vi "Updated Set Pointcycles.vi"(6 "Time2":T3, 8 "Time1":T2, 9 "rate":dbl, 10 "Amp":T1, 11 "i":i32) -> (12 "Gain times":cluster{dbl, dbl, dbl, dbl, dbl, dbl}, 13 "y":dbl)   [LabVIEW 2011]
panel:
  out "I tot":dbl
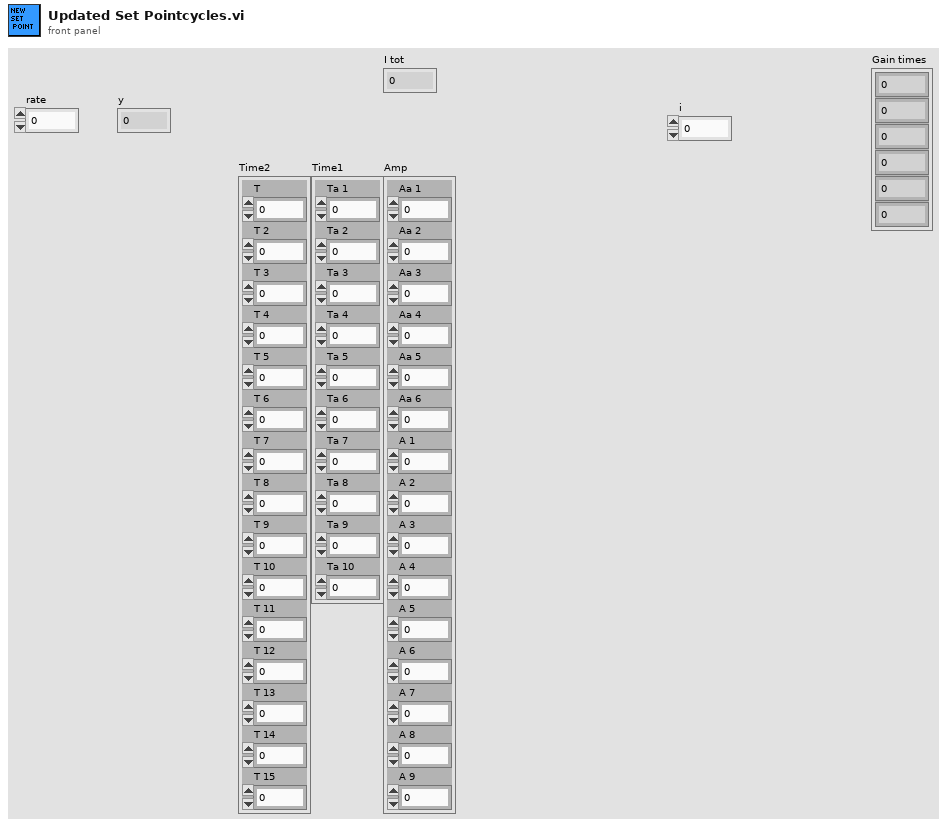
[diagram p1: front panel]
types:
  T1 = cluster{"Aa 1":dbl, "Aa 2":dbl, "Aa 3":dbl, "Aa 4":dbl, "Aa 5":dbl, "Aa 6":dbl, "A 1":dbl, "A 2":dbl, "A 3":dbl, "A 4":dbl, "A 5":dbl, "A 6":dbl, "A 7":dbl, "A 8":dbl, "A 9":dbl}
  T2 = cluster{"Ta 1":dbl, "Ta 2":dbl, "Ta 3":dbl, "Ta 4":dbl, "Ta 5":dbl, "Ta 6":dbl, "Ta 7":dbl, "Ta 8":dbl, "Ta 9":dbl, "Ta 10":dbl}
  T3 = cluster{"T":dbl, "T 2":dbl, "T 3":dbl, "T 4":dbl, "T 5":dbl, "T 6":dbl, "T 7":dbl, "T 8":dbl, "T 9":dbl, "T 10":dbl, "T 11":dbl, "T 12":dbl, "T 13":dbl, "T 14":dbl, "T 15":dbl}
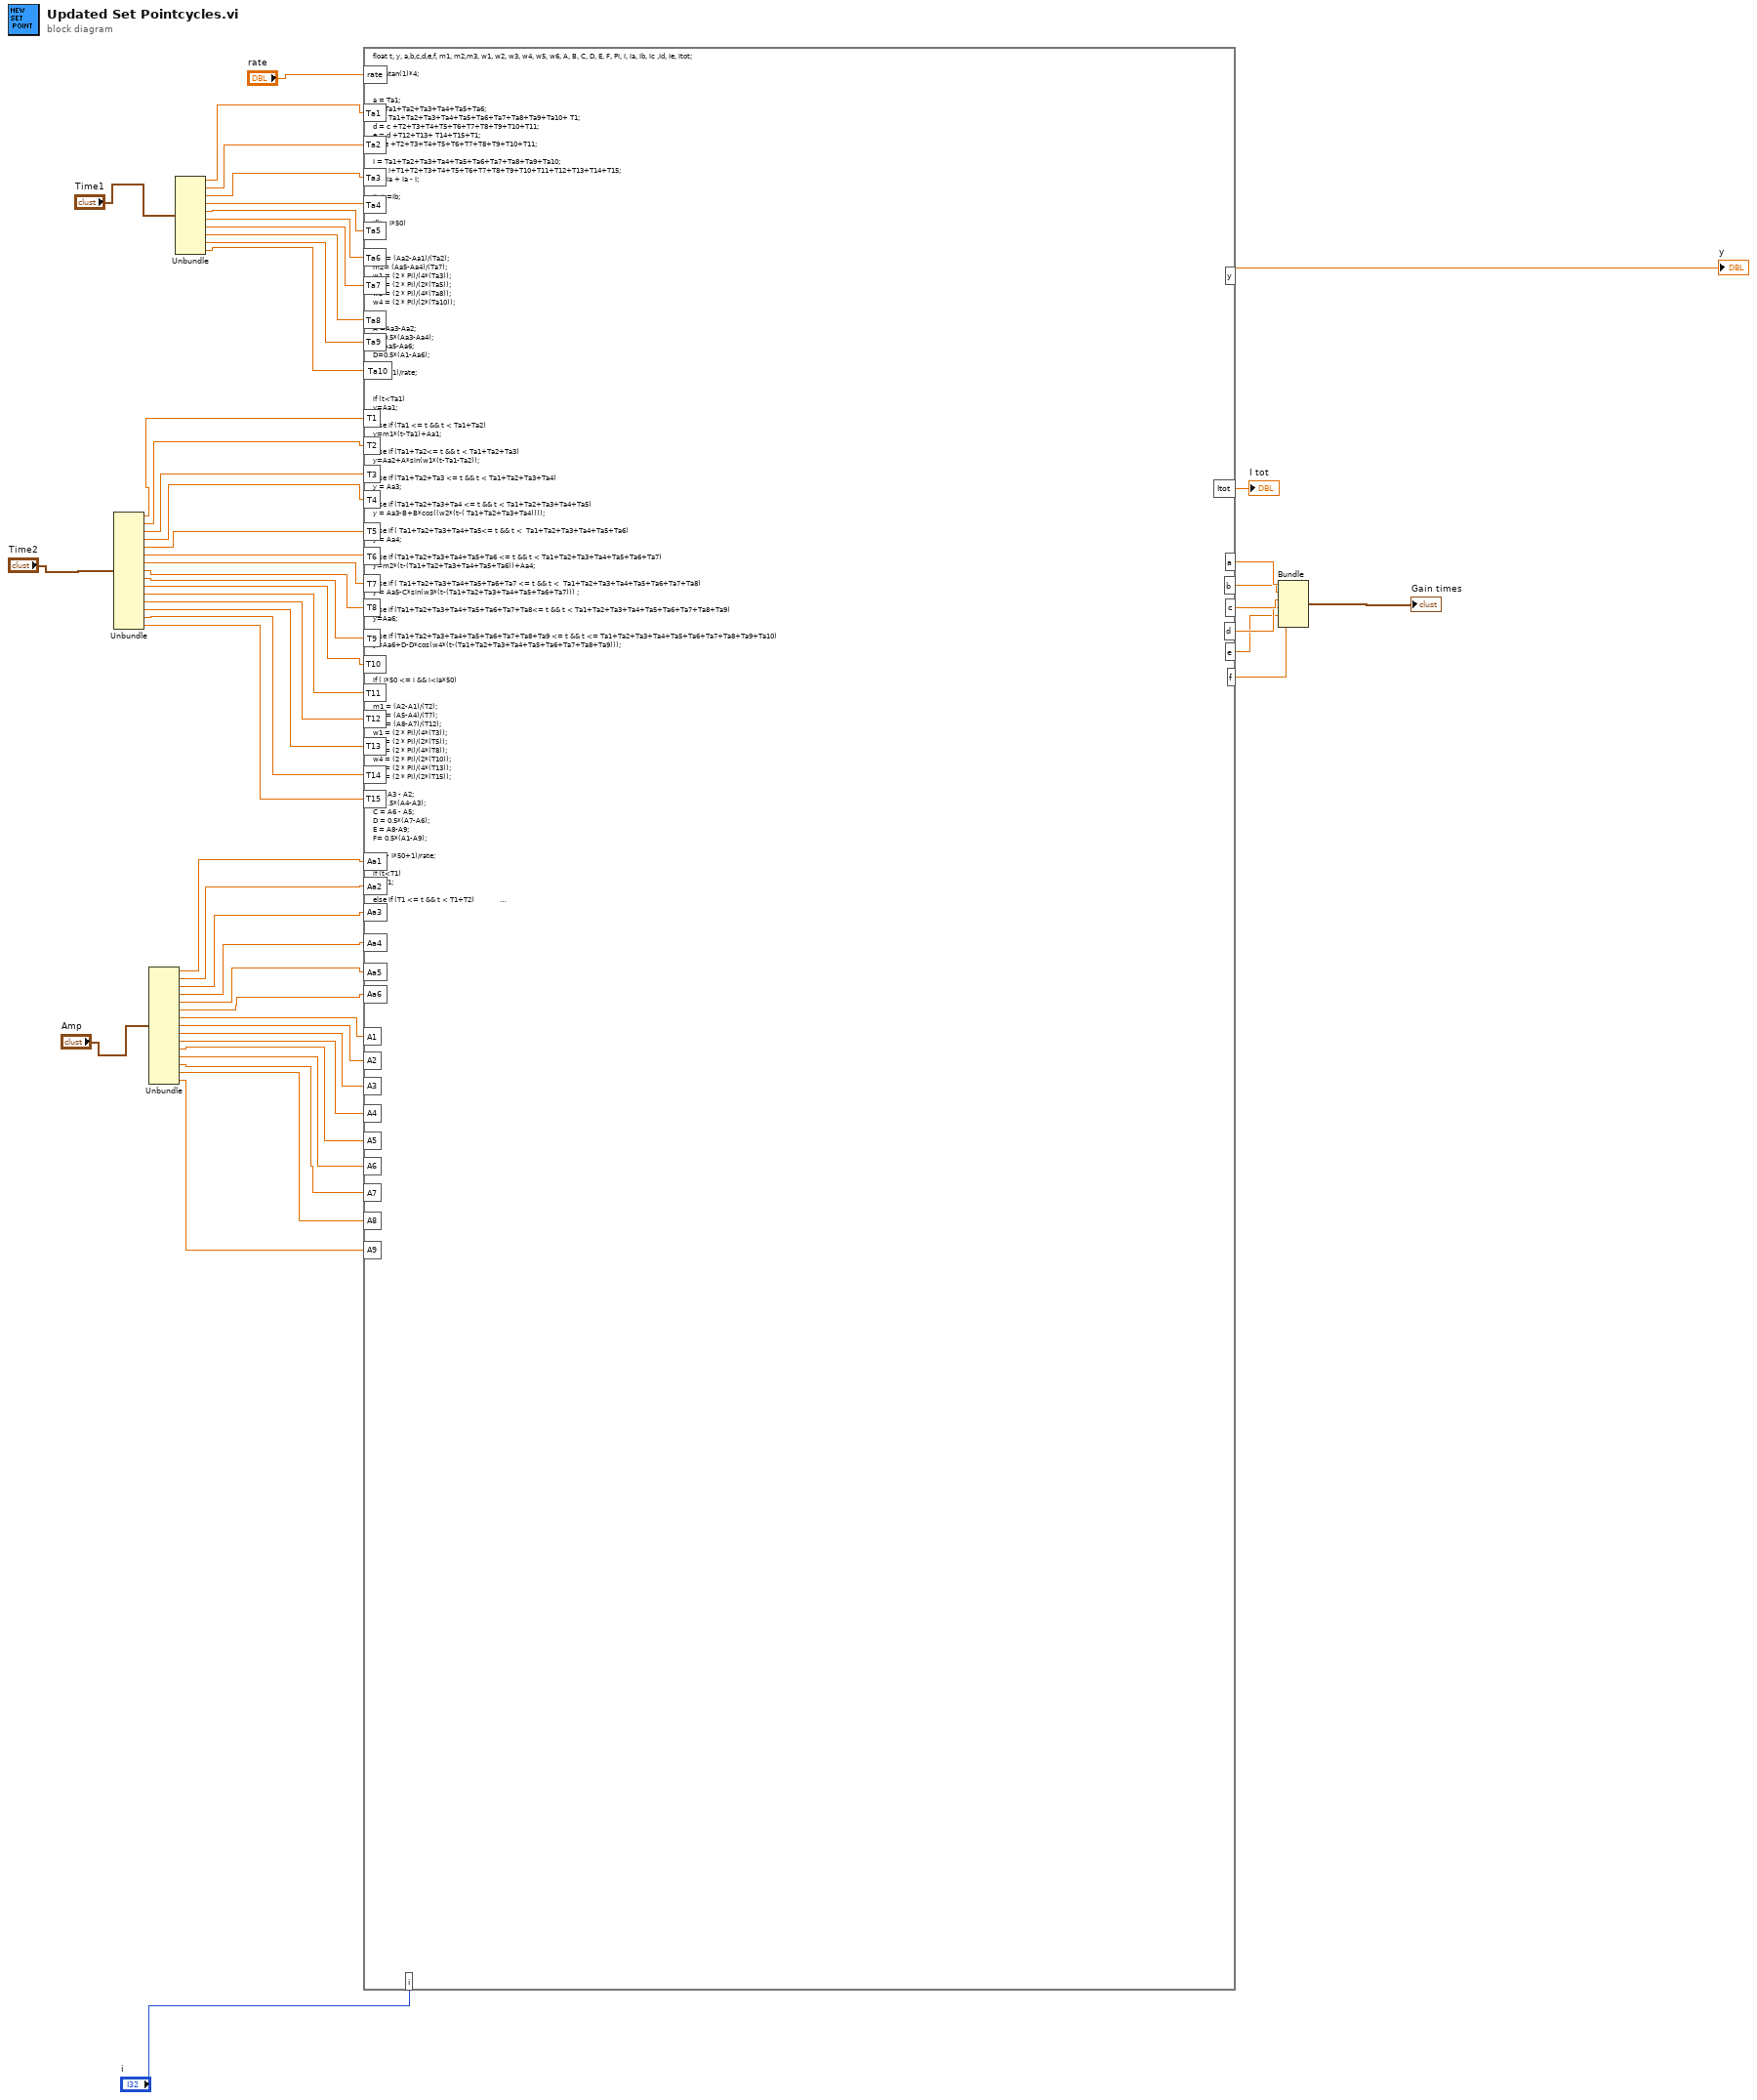
[diagram p0: block diagram]
diagram:
  n1 = Unbundle("Time2") -> ("T"=w43:dbl, "T 2"=w42:dbl, "T 3"=w41:dbl, "T 4"=w40:dbl, "T 5"=w39:dbl, "T 6"=w38:dbl, "T 7"=w37:dbl, "T 8"=w36:dbl, "T 9"=w35:dbl, "T 10"=w34:dbl, "T 11"=w33:dbl, "T 12"=w32:dbl, "T 13"=w31:dbl, "T 14"=w2:dbl, "T 15"=w1:dbl)
  n2 = Unbundle("Amp") -> ("Aa 1"=w20:dbl, "Aa 2"=w19:dbl, "Aa 3"=w18:dbl, "Aa 4"=w17:dbl, "Aa 5"=w16:dbl, "Aa 6"=w15:dbl, "A 1"=w14:dbl, "A 2"=w13:dbl, "A 3"=w12:dbl, "A 4"=w11:dbl, "A 5"=w10:dbl, "A 6"=w9:dbl, "A 7"=w8:dbl, "A 8"=w7:dbl, "A 9"=w3:dbl)
  n3 = Unbundle("Time1") -> ("Ta 1"=w30:dbl, "Ta 2"=w29:dbl, "Ta 3"=w28:dbl, "Ta 4"=w27:dbl, "Ta 5"=w26:dbl, "Ta 6"=w25:dbl, "Ta 7"=w24:dbl, "Ta 8"=w23:dbl, "Ta 9"=w22:dbl, "Ta 10"=w21:dbl)
  n4 = formula code="float t, y, a,b,c,d,e,f, m1, m2,m3, w1, w2, w3, w4, w5, w6, A, B, C, D, E, F, PI, I, Ia, Ib, Ic ,Id, Ie, Itot;\n\nPI=atan(1)*4;\n\n\na = Ta1;\nb= Ta1+Ta2+Ta3+Ta4+Ta5+Ta6;\nc =  Ta1+Ta2+Ta3+Ta4+Ta5+Ta6+Ta7+Ta8+Ta9+Ta10+ T1;\nd = c +T2+T3+T4+T5+T6+T7+T8+T9+T10+T11;\ne = d +T12+T13+ T14+T15+T1;\nf = e +T2+T3+T4+T5+T6+T7+T8+T9+T10+T11;\n\nI = Ta1+Ta2+Ta3+Ta4+Ta5+Ta6+Ta7+Ta8+Ta9+Ta10;\nIa = I+T1+T2+T3+T4+T5+T6+T7+T8+T9+T10+T11+T12+T13+T14+T15;\nIb =Ia + Ia - I;\n\nItot =Ib;\n\n\nif(i< I*50)\n{\n\n\nm1 = (Aa2-Aa1)/(Ta2);\nm2= (Aa5-Aa4)/(Ta7);\nw1 = (2 * PI)/(4*(Ta3));\nw2 = (2 * PI)/(2*(Ta5));\nw3 = (2 * PI)/(4*(Ta8));\nw4 = (2 * PI)/(2*(Ta10));\n\n\nA =Aa3-Aa2;\nB=0.5*(Aa3-Aa4);\nC=Aa5-Aa6;\nD=0.5*(A1-Aa6);\n\nt=(i+1)/rate;\n\n\nif (t<Ta1)\ny=Aa1;\n\nelse if (Ta1 <= t && t < Ta1+Ta2)\ny=m1*(t-Ta1)+Aa1;\n\nelse if (Ta1+Ta2<= t && t < Ta1+Ta2+Ta3)\ny=Aa2+A*sin(w1*(t-Ta1-Ta2));\n\nelse if (Ta1+Ta2+Ta3 <= t && t < Ta1+Ta2+Ta3+Ta4)\ny = Aa3;\n\nelse if (Ta1+Ta2+Ta3+Ta4 <= t && t < Ta1+Ta2+Ta3+Ta4+Ta5)\ny = Aa3-B+B*cos((w2*(t-( Ta1+Ta2+Ta3+Ta4))));\n\nelse if ( Ta1+Ta2+Ta3+Ta4+Ta5<= t && t <  Ta1+Ta2+Ta3+Ta4+Ta5+Ta6)\ny = Aa4;\n\nelse if (Ta1+Ta2+Ta3+Ta4+Ta5+Ta6 <= t && t < Ta1+Ta2+Ta3+Ta4+Ta5+Ta6+Ta7)\ny=m2*(t-(Ta1+Ta2+Ta3+Ta4+Ta5+Ta6))+Aa4;\n\nelse if ( Ta1+Ta2+Ta3+Ta4+Ta5+Ta6+Ta7 <= t && t <  Ta1+Ta2+Ta3+Ta4+Ta5+Ta6+Ta7+Ta8)\ny = Aa5-C*sin(w3*(t-(Ta1+Ta2+Ta3+Ta4+Ta5+Ta6+Ta7))) ;\n\nelse if (Ta1+Ta2+Ta3+Ta4+Ta5+Ta6+Ta7+Ta8<= t && t < Ta1+Ta2+Ta3+Ta4+Ta5+Ta6+Ta7+Ta8+Ta9)\ny=Aa6;\n\nelse if (Ta1+Ta2+Ta3+Ta4+Ta5+Ta6+Ta7+Ta8+Ta9 <= t && t <= Ta1+Ta2+Ta3+Ta4+Ta5+Ta6+Ta7+Ta8+Ta9+Ta10)\ny=Aa6+D-D*cos(w4*(t-(Ta1+Ta2+Ta3+Ta4+Ta5+Ta6+Ta7+Ta8+Ta9)));\n\n}\n\nif ( I*50 <= i && i<Ia*50)\n{\n\nm1 = (A2-A1)/(T2);\nm2 = (A5-A4)/(T7);\nm3 = (A8-A7)/(T12);\nw1 = (2 * PI)/(4*(T3));\nw2 = (2 * PI)/(2*(T5));\nw3 = (2 * PI)/(4*(T8));\nw4 = (2 * PI)/(2*(T10));\nw5 = (2 * PI)/(4*(T13));\nw6 = (2 * PI)/(2*(T15));\n\nA = A3 - A2;\nB = .5*(A4-A3);\nC = A6 - A5;\nD = 0.5*(A7-A6);\nE = A8-A9;\nF= 0.5*(A1-A9);\n\nt=(i- I*50+1)/rate;\n\nif (t<T1)\ny=A1;\n\nelse if (T1 <= t && t < T1+T2)              //First slope\ny=m1*(t-T1)+A1;\n\nelse if (T1+T2<= t && t < T1+T2+T3)         //First Upwardcosine\ny=A2+A*sin(w1*(t-T1-T2));\n\nelse if (T1+T2+T3 <= t && t < T1+T2+T3+T4)    //First plateau\ny = A3;\n\nelse if ( T1+T2+T3+T4 <= t && t <  T1+T2+T3+T4+T5)    //first downward cosine  \ny = A3+B-B*cos((w2*(t-( T1+T2+T3+T4))));\n\nelse if ( T1+T2+T3+T4+T5<= t && t <  T1+T2+T3+T4+T5+T6)   //Second Plateau  \ny=A4;\n\nelse if (T1+T2+T3+T4+T5+T6 <= t && t < T1+T2+T3+T4+T5+T6+T7) // second slope  \ny=m2*(t-(T1+T2+T3+T4+T5+T6))+A4;\n\n\nelse if ( T1+T2+T3+T4+T5+T6+T7 <= t && t <  T1+T2+T3+T4+T5+T6+T7+T8)   //Second Upwardcosine     \ny=A5+C*sin(w3*(t-(T1+T2+T3+T4+T5+T6+T7)));\n\nelse if (T1+T2+T3+T4+T5+T6+T7+T8<= t && t < T1+T2+T3+T4+T5+T6+T7+T8+T9)  //Third Plateau\ny = A6;\n\nelse if (T1+T2+T3+T4+T5+T6+T7+T8+T9 <= t && t <= T1+T2+T3+T4+T5+T6+T7+T8+T9+T10)    //second downward cosine  \ny = A6+D-D*cos((w4*(t-( T1+T2+T3+T4+T5+T6+T7+T8+T9))));\n\nelse if (T1+T2+T3+T4+T5+T6+T7+T8+T9+T10 <= t && t <= T1+T2+T3+T4+T5+T6+T7+T8+T9+T10+T11) // Fourth plateau\ny=A7;\n\nelse if (T1+T2+T3+T4+T5+T6+T7+T8+T9+T10+T11 <= t && t <= T1+T2+T3+T4+T5+T6+T7+T8+T9+T10+T11+T12)\ny=m3*(t-(T1+T2+T3+T4+T5+T6+T7+T8+T9+T10+T11))+A7;          //downward slope     \n\n\nelse if (T1+T2+T3+T4+T5+T6+T7+T8+T9+T10+T11+T12 <= t && t <= T1+T2+T3+T4+T5+T6+T7+T8+T9+T10+T11+T12+T13)\ny = A8-E*sin(w5*(t-(T1+T2+T3+T4+T5+T6+T7+T8+T9+T10+T11+T12))) ; // downward cosine after linear slope \n\n\nelse if (T1+T2+T3+T4+T5+T6+T7+T8+T9+T10+T11+T12+T13 <= t && t <= T1+T2+T3+T4+T5+T6+T7+T8+T9+T10+T11+T12+T13+T14)\ny = A9;                             // Fifth Plateau\n \nelse if (T1+T2+T3+T4+T5+T6+T7+T8+T9+T10+T11+T12+T13+T14 <= t && t <= T1+T2+T3+T4+T5+T6+T7+T8+T9+T10+T11+T12+T13+T14+T15)\ny=A9+F-F*cos(w6*(t-(T1+T2+T3+T4+T5+T6+T7+T8+T9+T10+T11+T12+T13+T14)));   //Last upward cosine\n}\n\n\n\nif ( Ia*50 <= i )\n{\n\nm1 = (A2-A1)/(T2);\nm2 = (A5-A4)/(T7);\nm3 = (A8-A7)/(T12);\nw1 = (2 * PI)/(4*(T3));\nw2 = (2 * PI)/(2*(T5));\nw3 = (2 * PI)/(4*(T8));\nw4 = (2 * PI)/(2*(T10));\nw5 = (2 * PI)/(4*(T13));\nw6 = (2 * PI)/(2*(T15));\n\nA = A3 - A2;\nB = .5*(A4-A3);\nC = A6 - A5;\nD = 0.5*(A7-A6);\nE = A8-A9;\nF = 0.5*(A1-A9);\n\nt=(i- Ia*50+1)/rate;\n\nif (t<T1)\ny=A1;\n\nelse if (T1 <= t && t < T1+T2)              //First slope\ny=m1*(t-T1)+A1;\n\nelse if (T1+T2<= t && t < T1+T2+T3)         //First Upwardcosine\ny=A2+A*sin(w1*(t-T1-T2));\n\nelse if (T1+T2+T3 <= t && t < T1+T2+T3+T4)    //First plateau\ny = A3;\n\nelse if ( T1+T2+T3+T4 <= t && t <  T1+T2+T3+T4+T5)    //first downward cosine  \ny = A3+B-B*cos((w2*(t-( T1+T2+T3+T4))));\n\nelse if ( T1+T2+T3+T4+T5<= t && t <  T1+T2+T3+T4+T5+T6)   //Second Plateau  \ny=A4;\n\nelse if (T1+T2+T3+T4+T5+T6 <= t && t < T1+T2+T3+T4+T5+T6+T7) // second slope  \ny=m2*(t-(T1+T2+T3+T4+T5+T6))+A4;\n\n\nelse if ( T1+T2+T3+T4+T5+T6+T7 <= t && t <  T1+T2+T3+T4+T5+T6+T7+T8)   //Second Upwardcosine     \ny=A5+C*sin(w3*(t-(T1+T2+T3+T4+T5+T6+T7)));\n\nelse if (T1+T2+T3+T4+T5+T6+T7+T8<= t && t < T1+T2+T3+T4+T5+T6+T7+T8+T9)  //Third Plateau\ny = A6;\n\nelse if (T1+T2+T3+T4+T5+T6+T7+T8+T9 <= t && t <= T1+T2+T3+T4+T5+T6+T7+T8+T9+T10)    //second downward cosine  \ny = A6+D-D*cos((w4*(t-( T1+T2+T3+T4+T5+T6+T7+T8+T9))));\n\nelse if (T1+T2+T3+T4+T5+T6+T7+T8+T9+T10 <= t && t <= T1+T2+T3+T4+T5+T6+T7+T8+T9+T10+T11) // Fourth plateau\ny=A7;\n\nelse if (T1+T2+T3+T4+T5+T6+T7+T8+T9+T10+T11 <= t && t <= T1+T2+T3+T4+T5+T6+T7+T8+T9+T10+T11+T12)\ny=m3*(t-(T1+T2+T3+T4+T5+T6+T7+T8+T9+T10+T11))+A7;          //downward slope     \n\n\nelse if (T1+T2+T3+T4+T5+T6+T7+T8+T9+T10+T11+T12 <= t && t <= T1+T2+T3+T4+T5+T6+T7+T8+T9+T10+T11+T12+T13)\ny = A8-E*sin(w5*(t-(T1+T2+T3+T4+T5+T6+T7+T8+T9+T10+T11+T12))) ; // downward cosine after linear slope \n\n\nelse if (T1+T2+T3+T4+T5+T6+T7+T8+T9+T10+T11+T12+T13 <= t && t <= T1+T2+T3+T4+T5+T6+T7+T8+T9+T10+T11+T12+T13+T14)\ny = A9;                             // Fifth Plateau\n \nelse if (T1+T2+T3+T4+T5+T6+T7+T8+T9+T10+T11+T12+T13+T14 <= t && t <= T1+T2+T3+T4+T5+T6+T7+T8+T9+T10+T11+T12+T13+T14+T15)\ny=A9+F-F*cos(w6*(t-(T1+T2+T3+T4+T5+T6+T7+T8+T9+T10+T11+T12+T13+T14)));   //Last upward cosine\n}"("i"="i", "rate"="rate", "Ta1"=w30, "Ta2"=w29, "Ta3"=w28, "Ta4"=w27, "Ta5"=w26, "Ta6"=w25, "Ta7"=w24, "Ta8"=w23, "Ta9"=w22, "Ta10"=w21, "T1"=w43, "T2"=w42, "T3"=w41, "T4"=w40, "T5"=w39, "T6"=w38, "T7"=w37, "T8"=w36, "T9"=w35, "T10"=w34, "T11"=w33, "T12"=w32, "T13"=w31, "Aa1"=w20, "Aa2"=w19, "Aa3"=w18, "Aa4"=w17, "Aa5"=w16, "Aa6"=w15, "A1"=w14, "A2"=w13, "A3"=w12, "A4"=w11, "A5"=w10, "A6"=w9, "A7"=w8, "A8"=w7, "T15"=w1, "T14"=w2, "A9"=w3) -> ("y"=→"y":dbl, "Itot"=→"I tot":dbl, "a"=w51:dbl, "b"=w50:dbl, "c"=w49:dbl, "d"=w48:dbl, "e"=w47:dbl, "f"=w46:dbl)
  n5 = Bundle(w51, w50, w49, w48, w47, w46) -> (→"Gain times":cluster{dbl, dbl, dbl, dbl, dbl, dbl})  [unwired: 1 in]
